vi "User Console View.vi"(8 "error in (no error)":errorcluster, 11 "View Model":T1) -> (0 "error out":errorcluster)   [LabVIEW 2017]
doc: "The interface where a user calls the Elevator, makes a floor selection, and reports Emergency.\n[Covers: UI2]"
uses:
  View Model/Controls/View Model.ctl
  View Model/Controls/Shared Model.ctl
  Error Handler/Controls/Error Model.ctl
  Error Handler/Controls/Error Data.ctl
  Error Handler/Controls/Error Level.ctl
  Configuration/Controls/Config Model.ctl
  Configuration/Controls/Config Data Record.ctl
  Configuration/Controls/Config Command.ctl
  Controller/Controls/Control Model.ctl
  Controller/Controls/Elevator Location.ctl
  Controller/Controls/Elevator Status.ctl
  Controller/Controls/Control Event.ctl
  Controller/Controls/Control CMD.ctl
  Controller/Controls/Controller - Overhead.ctl
  Controls/User Console - References.ctl
  Controller/Controls/Timer Commands.ctl
panel:
  in  "Emergency":bool
  in  "Close Door":bool
  in  "Open Door":bool
  in  "1st Floor":bool
  in  "2nd Floor":bool
  in  "3rd Floor":bool
  in  "4th Floor":bool
  in  "2nd Down":bool
  in  "3rd Down":bool
  in  "4th Down":bool
  in  "3rd Up":bool
  in  "2nd Up":bool
  in  "1st Up":bool
  # "Elevator Call"
  # "Floor Selection"
  # "[Covers: UI2B2]"
  # "[Covers: UI2A]"
  # "[Covers: UI2A1]"
  # "[Covers: UI2A2]"
  # "[Covers: UI2B]"
  # "Door Buttons"
  # "[Covers: UI2C]"
  # "[Covers: UI2D]"
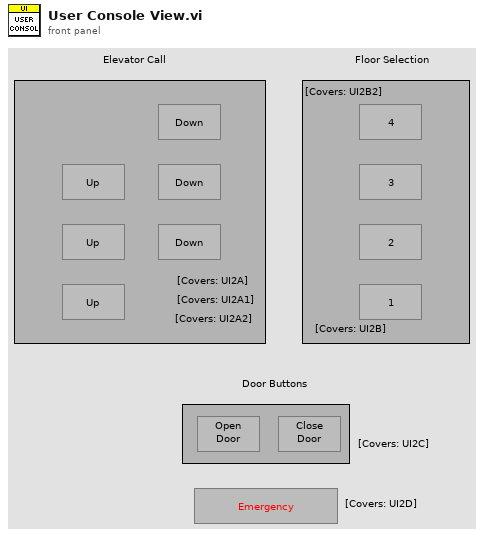
[diagram p1: front panel]
types:
  T1 = typedef "View Model.ctl" = cluster{"Shared Model":T2, "Error Model":T3, "Config Model":T4, "Control Model":T5}
  T2 = typedef "Shared Model.ctl" = cluster{"Stop":refnum<user-event>, "Stop DVR":refnum<data-value>}
  T3 = typedef "Error Model.ctl" = cluster{"Error":refnum<user-event>}
  T4 = typedef "Config Model.ctl" = cluster{"Data DVR":refnum<data-value>, "Config CMD":refnum<user-event>}
  T5 = typedef "Control Model.ctl" = cluster{"Location Change":refnum<user-event>, "Direction Change":refnum<user-event>, "Door Posit Change":refnum<user-event>, "Emergency Change":refnum<user-event>, "Status Change":refnum<user-event>, "Command":refnum<user-event>, "Overhaed DVR":refnum<data-value>}
  T6 = typedef "Elevator Status.ctl" = enum16{"No Request", "Initial", "Wait for 1st Request", "Start and Move", "Continue Move", "Analysis", "Stop at Floor", "Open/Close Door", "Emergency Call", "Terminate"}
  T7 = typedef "User Console - References.ctl" = cluster{"Open Door":refnum<vi>, "Close Door":refnum<vi>, "Emergency":refnum<vi>, "1st Up":refnum<vi>, "2nd Up":refnum<vi>, "3rd Up":refnum<vi>, "2nd Down":refnum<vi>, "3rd Down":refnum<vi>, "4th Down":refnum<vi>}
  T8 = typedef "Control CMD.ctl" = enum16{"Idle", "Call", "Go Up", "Go Down", "Go to Floor", "Open Door", "Close Door", "Emergency"}
  T9 = typedef "Timer Commands.ctl" = enum16{"Start", "Restart", "Get", "Pause"}
  T10 = enum8{"Enabled", "Disabled", "Disabled and Grayed Out"}
  T11 = typedef "Elevator Location.ctl" = enum16{"1st Floor", "2nd Floor", "3rd Floor", "4th Floor"}
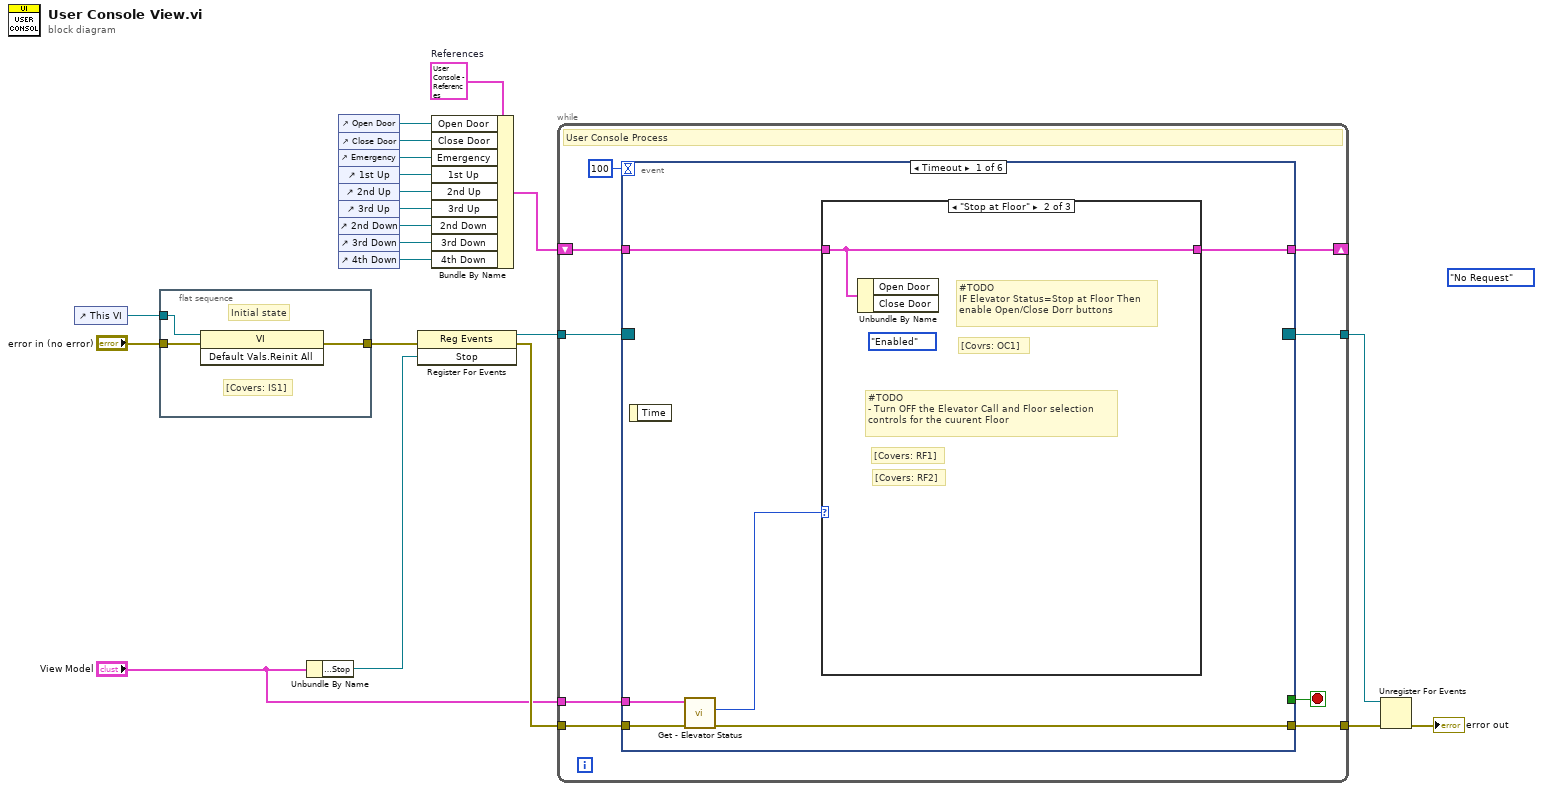
[diagram p0: block diagram]
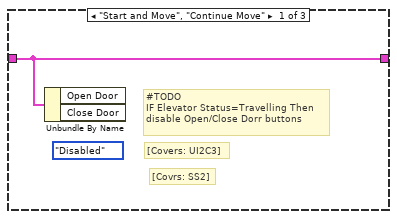
[diagram p2: hidden frame]
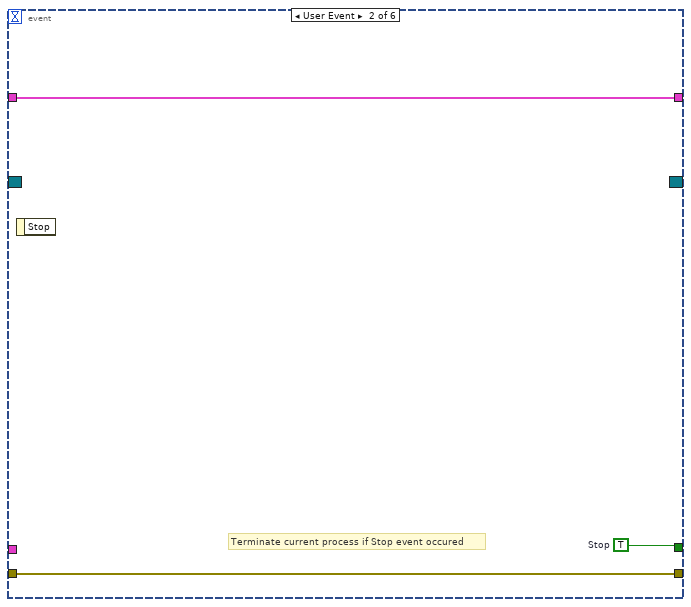
[diagram p4: hidden frame]
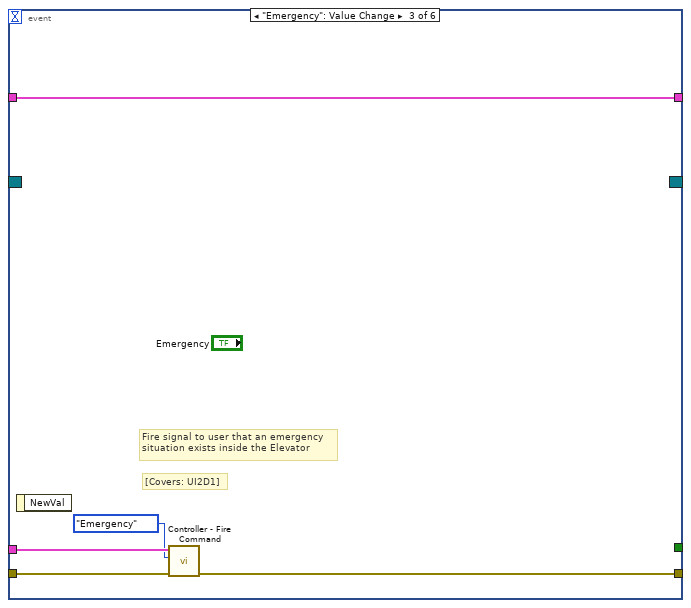
[diagram p5: hidden frame]
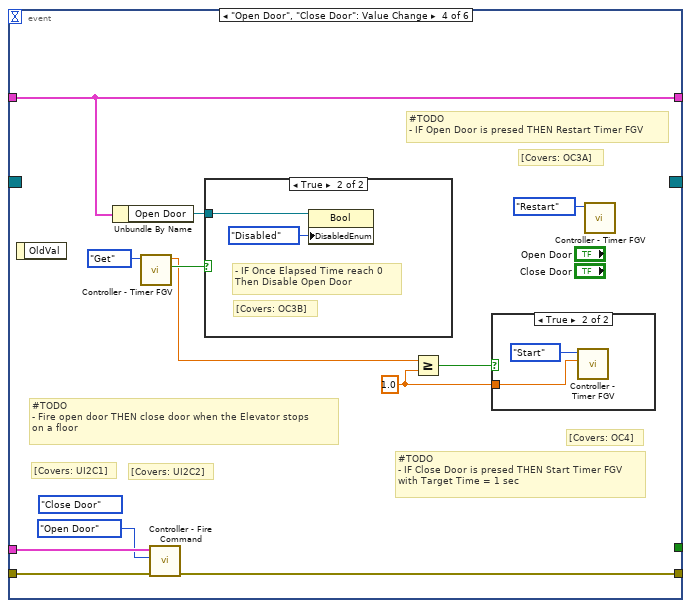
[diagram p6: hidden frame]
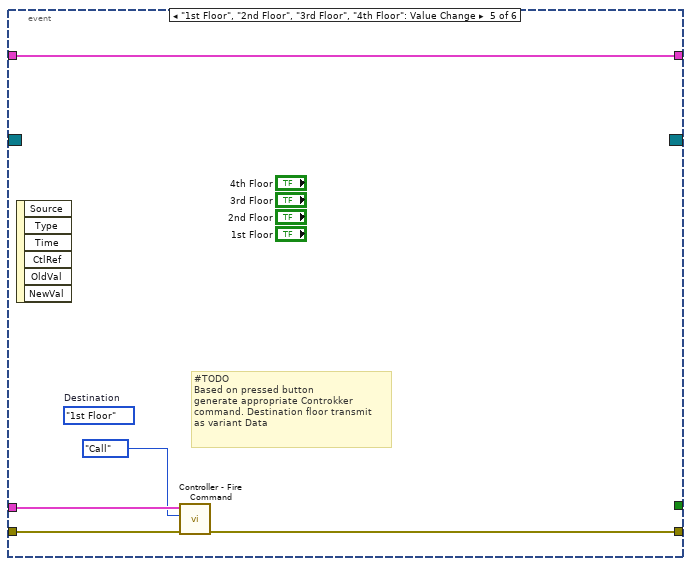
[diagram p9: hidden frame]
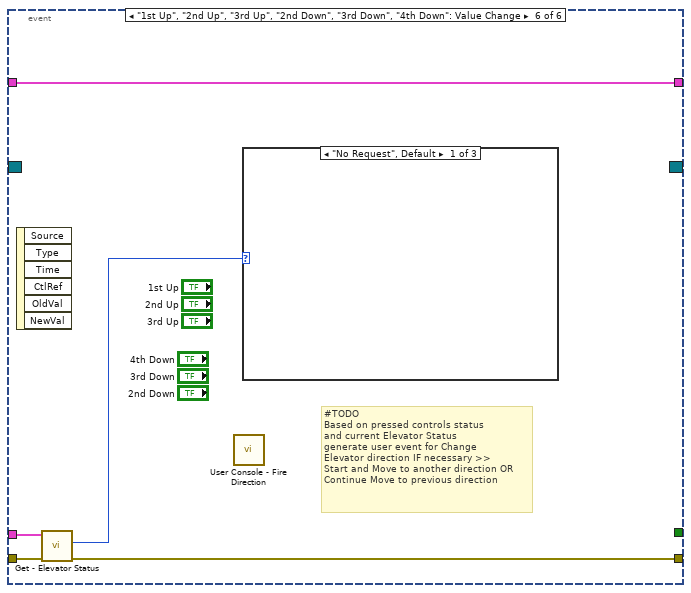
[diagram p10: hidden frame]
diagram:
  (unwired) Elevator_Status."No Request" ("Elevator Status")
  w14 = T7 {"Open Door"=refnum, "Close Door"=refnum, "Emergency"=refnum, "1st Up"=refnum, "2nd Up"=refnum, "3rd Up"=refnum, "2nd Down"=refnum, "3rd Down"=refnum, "4th Down"=refnum}  # References
  n1 = control-ref of="This VI"() -> (w1:refnum<vi>)
  n2 = flat-sequence {
    tunnel: "error in (no error)" -> [w24]
    tunnel: [w23] -> w2
    tunnel: w1 -> [w22]
    frame #0 {
      # "[Covers: IS1]"
      # "Initial state"
      n3 = invoke class="VI" method="Default Vals.Reinit All"(reference=w22, error in=w24) -> (error out=w23:errorcluster)  [unwired: 1 in, 2 out]
    }
  }
  n4 = Unbundle By Name("View Model") -> ("Shared Model.Stop"=w21:refnum<user-event>)
  n5 = control-ref of="Open Door"() -> (w13:refnum<vi>)
  n6 = control-ref of="Close Door"() -> (w11:refnum<vi>)
  n7 = control-ref of="Emergency"() -> (w10:refnum<vi>)
  n8 = control-ref of="1st Up"() -> (w9:refnum<vi>)
  n9 = control-ref of="2nd Up"() -> (w8:refnum<vi>)
  n10 = control-ref of="3rd Up"() -> (w7:refnum<vi>)
  n11 = control-ref of="2nd Down"() -> (w6:refnum<vi>)
  n12 = control-ref of="3rd Down"() -> (w5:refnum<vi>)
  n13 = control-ref of="4th Down"() -> (w12:refnum<vi>)
  n14 = register-events(error in=w2, w21) -> (reference out=w20:refnum<event-registration>, error out=w19:errorcluster)  [unwired: 1 in]
  n15 = Bundle By Name(cluster=w14, "Open Door"=w13, "Close Door"=w11, "Emergency"=w10, "1st Up"=w9, "2nd Up"=w8, "3rd Up"=w7, "2nd Down"=w6, "3rd Down"=w5, "4th Down"=w12) -> (w4:T7)
  n16 = while {
    tunnel: w20 -> [w33]
    tunnel: w19 -> [w32]
    tunnel: [w31] -> w17
    tunnel: [w29] -> w18
    tunnel: "View Model" -> [w28]
    shift-right: [w25] -> _
    shift-left: w4 -> [w26]
    stop <- w30 stop-if-true
    # "User Console Process"
    n17 = event shown="[0] Timeout" {
      selector: w33 -> [_ _ _ _ _ _]
      dyn-events: [_ _ _ _ _ _] -> w29
      timeout: 100 -> [_ _ _ _ _ _]
      tunnel: w32 -> [w39 w45 w49 w62 w70 w75]
      tunnel: [w37 w45 w48 w61 w69 w72] -> w31
      tunnel: [_ w44 _ _ _ _] -> w30
      tunnel: w28 -> [w38 _ w47 w60 w68 w74]
      tunnel: w26 -> [w35 w43 w50 w55 w71 w76]
      tunnel: [w34 w43 w50 w55 w71 w76] -> w25
      event Timeout {
        n18 = event-data() -> ()  [unwired: 1 in, 1 out]
        n19 = call "Get - Elevator Status.vi"("error in (no error)"=w39, "View Model"=w38) -> ("error out"=w37:errorcluster, "Current Status"=w36:T6)  [unwired: 6 in, 2 out]
        n20 = case shown="\"Stop at Floor\"" w36 {
          tunnel: w35 -> [w40 w41 w42]
          tunnel: [w40 w41 w42] -> w34
          frame "Start and Move", "Continue Move" {
            (unwired) T10."Disabled" ("Disabled")
            # "[Covrs: SS2]"
            # "[Covers: UI2C3]"
            # "#TODO\nIF Elevator Status=Travelling Then \ndisable Open/Close Dorr buttons"
            n21 = Unbundle By Name(w40) -> ()  [unwired: 2 out]
          }
          frame "Stop at Floor" {
            (unwired) T10."Enabled" ("Disabled")
            # "[Covers: RF2]"
            # "[Covers: RF1]"
            # "#TODO\n- Turn OFF the Elevator Call and Floor selection\ncontrols for the cuurent Floor"
            # "[Covrs: OC1]"
            # "#TODO\nIF Elevator Status=Stop at Floor Then \nenable Open/Close Dorr buttons"
            n22 = Unbundle By Name(w41) -> ()  [unwired: 2 out]
          }
          frame "No Request", Default {
          }
        }
      }
      event User Event {
        w44 = TRUE  # Stop
        # "Terminate current process if Stop event occured"
        n23 = event-data() -> ()  [unwired: 1 in, 1 out]
      }
      event "Emergency": Value Change {
        # "[Covers: UI2D1]"
        # "Fire signal to user that an emergency\nsituation exists inside the Elevator"
        n24 = event-data() -> ()  [unwired: 1 in, 1 out]
        n25 = call "Controller - Fire Command.vi"("error in (no error)"=w49, "CMD"=Control_CMD."Emergency", "View Model"=w47) -> ("error out"=w48:errorcluster)  [unwired: 7 in, 1 out]
      }
      event "Open Door", "Close Door": Value Change {
        w51 = 1.0 ("Target Time. s")
        (unwired) Control_CMD."Close Door" ("CMD")
        # "[Covers: OC4]"
        # "#TODO\n- IF Close Door is presed THEN Start Timer FGV\nwith Target Time = 1 sec"
        # "[Covers: OC3A]"
        # "#TODO\n- IF Open Door is presed THEN Restart Timer FGV"
        # "[Covers: UI2C2]"
        # "[Covers: UI2C1]"
        # "#TODO\n- Fire open door THEN close door when the Elevator stops\non a floor"
        n26 = event-data() -> ()  [unwired: 1 in, 1 out]
        n27 = Unbundle By Name(w55) -> ("Open Door"=w54:refnum<vi>)
        n28 = call "Controller - Timer FGV.vi"("Timer CMD"=Timer_Commands."Get") -> ("Elapsed?"=w56:bool, "Elapsed Time"=w53:dbl)  [unwired: 8 in, 1 out]
        n29 = call "Controller - Fire Command.vi"("error in (no error)"=w62, "CMD"=Control_CMD."Open Door", "View Model"=w60) -> ("error out"=w61:errorcluster)  [unwired: 7 in, 1 out]
        n30 = case shown="True" w56 {
          tunnel: w54 -> [_ w66]
          frame False {
          }
          frame True {
            # "[Covers: OC3B]"
            # "- IF Once Elapsed Time reach 0 \nThen Disable Open Door"
            n31 = property class="Bool"(reference=w66, "DisabledEnum"=T10."Disabled" ("Disabled")) -> ()  [unwired: 1 in, 2 out]
          }
        }
        n32 = Greater Or Equal?(x=w53, y=w51) -> (x >= y?=w52:bool)
        n33 = case shown="True" w52 {
          tunnel: w51 -> [_ w63]
          frame False {
          }
          frame True {
            n34 = call "Controller - Timer FGV.vi"("Target Time. s"=w63, "Timer CMD"=Timer_Commands."Start") -> ()  [unwired: 7 in, 3 out]
          }
        }
        n35 = call "Controller - Timer FGV.vi"("Timer CMD"=Timer_Commands."Restart") -> ()  [unwired: 8 in, 3 out]
      }
      event "1st Floor", "2nd Floor", "3rd Floor", "4th Floor": Value Change {
        (unwired) Elevator_Location."1st Floor"  # Destination
        # "#TODO\nBased on pressed button\ngenerate appropriate Controkker\ncommand. Destination floor transmit\nas variant Data"
        n36 = event-data() -> ()  [unwired: 1 in, 6 out]
        n37 = call "Controller - Fire Command.vi"("error in (no error)"=w70, "CMD"=Control_CMD."Call", "View Model"=w68) -> ("error out"=w69:errorcluster)  [unwired: 7 in, 1 out]
      }
      event "1st Up", "2nd Up", "3rd Up", "2nd Down", "3rd Down", "4th Down": Value Change {
        # "#TODO\nBased on pressed controls status\nand current Elevator Status\ngenerate user event for Change \nElevator direction IF necessary >>\nStart and Move to another direction OR\nContinue Move to previous direction"
        n38 = event-data() -> ()  [unwired: 1 in, 6 out]
        n39 = call "Get - Elevator Status.vi"("error in (no error)"=w75, "View Model"=w74) -> ("error out"=w72:errorcluster, "Current Status"=w73:T6)  [unwired: 6 in, 2 out]
        n40 = call "User Console - Fire Direction.vi"() -> ()  [unwired: 10 in, 2 out]
        n41 = case shown="\"No Request\", Default" w73 {
          frame "No Request", Default {
          }
          frame "Start and Move" {
          }
          frame "Continue Move" {
          }
        }
      }
    }
  }
  n42 = Unregister For Events(event registration refnum=w18, error in=w17) -> (error out=→"error out":errorcluster)
